vi "30_Tasks on Array.vi"() -> ()   [LabVIEW 2018]
panel:
  out "Sub Array":dbl[](array[numeric])
  out "Array Scaled by 10":dbl[](array[numeric])
  out "Initial Array":dbl[](array[numeric])
  # "Build a VI that generates 1D array of 10 elements. Multiply the array\nelements by scaling factor of 10 and find the resultant array"
  # "Create a subset array of 5 elements from the resultant array."
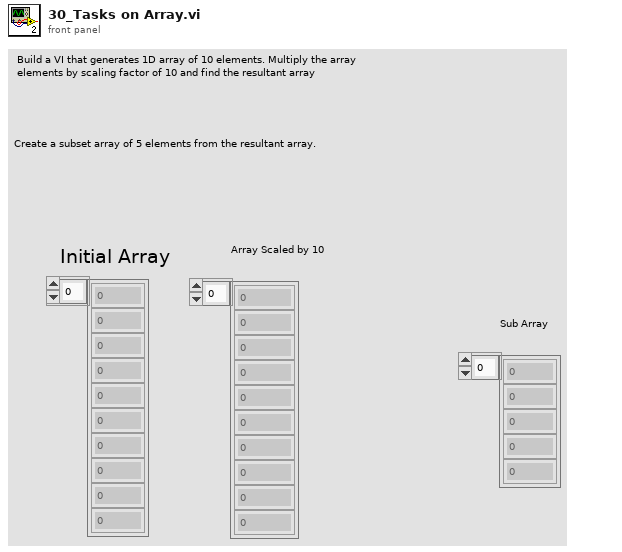
[diagram p1: front panel]
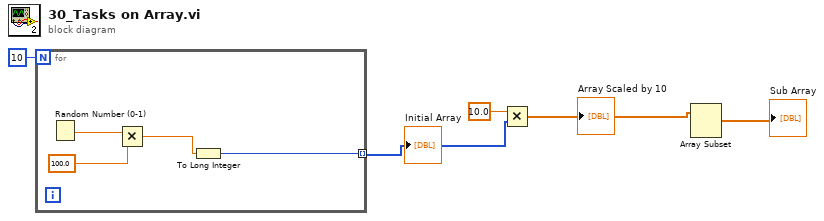
[diagram p0: block diagram]
diagram:
  n1 = for {
    N: 10 -> [_]
    tunnel: [w7] -> w3 mode=indexing
    n2 = Random Number (0-1)() -> (number: 0 to 1=w9:dbl)
    n3 = Multiply(x=w9, y=100.0 ("x")) -> (x*y=w8:dbl)
    n4 = To Long Integer(number=w8) -> (32bit integer=w7:i32)
  }
  "Initial Array" <- w3
  n5 = Multiply(x=10.0, y=w3) -> (x*y=w2:dbl[])
  "Array Scaled by 10" <- w2
  n6 = Array Subset(array=w2) -> (→"Sub Array":dbl[])  [unwired: 2 in]
